vi "Parse and Attach Metadata to TDMS.vi"(8 "error in (no error)":errorcluster, 11 "experiment folder":path) -> (0 "error out":errorcluster, 2 "file path out":path)   [LabVIEW 2016]
uses:
  <userlib>/_OpenG.lib/file/file.llb/Build Path - Traditional__ogtk.vi
  <userlib>/LevyLab/LV to ITX/Data/Data.lvclass
panel:
  out "wiring":string[][][](array[string])
  out "itx notes parsed iterations":i32
  out "Array":string[](array[string])
  out "group/channel names":string[][](array[string])
  out "group names":string[](array[string])
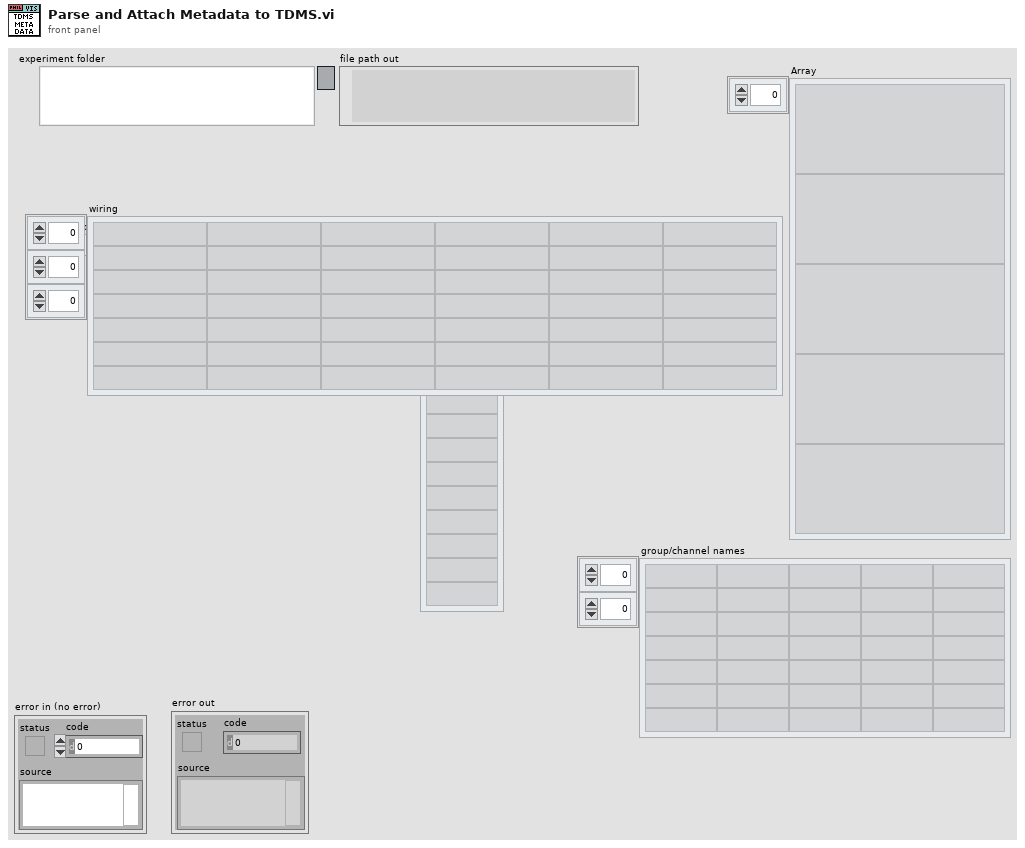
[diagram p1: front panel]
types:
  T1 = enum16{"open", "open or create", "create or replace", "create", "open (read-only)"}
  T2 = cluster{"Scan control":cluster{"Priority":enum16{"Priority 0", "Priority 1", "Priority 2", "Priority 3", "Priority 4", "Priority 5"}, "Scan name":enum16{"OFF", "DSA_Vsg2", "DSA_Vsg3", "DSA_Vbg", "DSA_Vsg1", "DSA_freq", "DSA_Vamp", "time", "Lockin Amplitude", "Lockin Frequency", "Lockin Bias", "Delay", "Strain", "DAQ Bias", "Magnet Field", "Temperature", "MW f1", "MW f2", "MW Amplitude1", "MW Amplitude2"}}[], "Scan parameters":cluster{"Start":dbl, "End":dbl, "Step":dbl, "Rate":dbl, "wait (ms)":u32, "Address":string, "channel":i32}[], "Experiment":enum16{"IV", "IV_Fast", "IV_Sweep", "THz_DelayLine", "Lockin_Vsg", "Lockin_Sweep", "Lockin_Time", "AI WFM time", "Lockin (experimental)"}}
  T3 = cluster{"AO Amp (V)":dbl[], "AO DC (V)":dbl[], "AO f (Hz)":dbl[], "AO Phase (°)":dbl[], "Function":enum16{"Sine", "Triangle", "Square", "Sawtooth"}[], "I+":bool[], "Sweeping":bool[]}
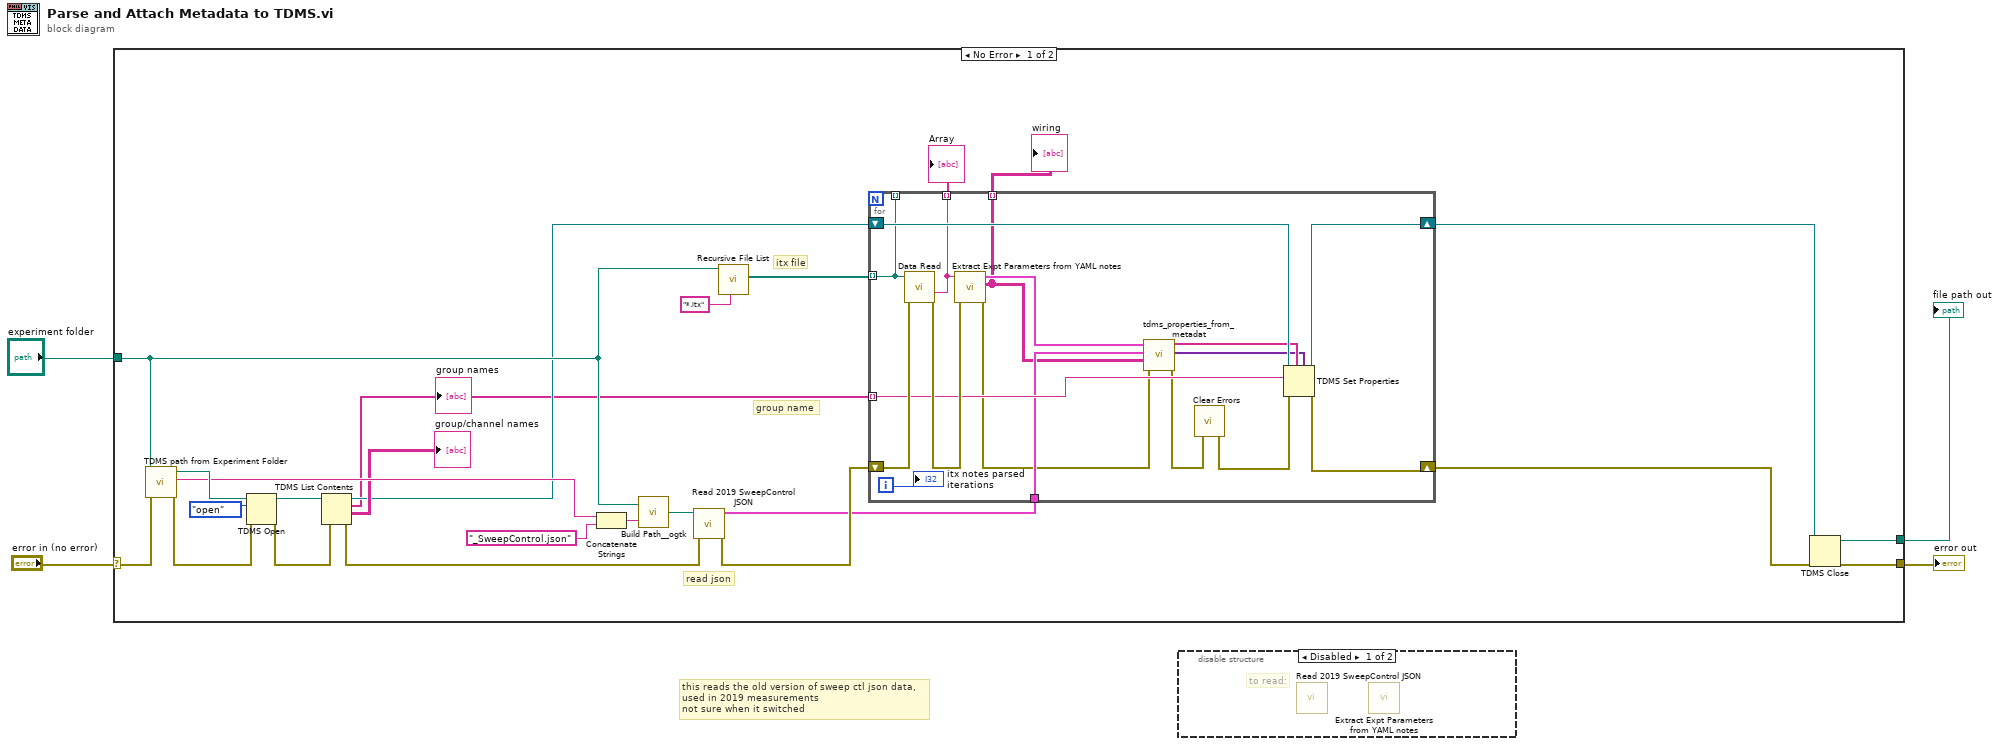
[diagram p0: block diagram]
diagram:
  # "this reads the old version of sweep ctl json data,\nused in 2019 measurements\nnot sure when it switched"
  n1 = case shown="No Error" "error in (no error)" {
    selector: "error in (no error)" -> [w25 w47]
    tunnel: [w12 w47] -> w3
    tunnel: "experiment folder" -> [w22 _]
    tunnel: [w11 _] -> w1
    frame No Error {
      # "itx file"
      # "group name"
      # "read json"
      n2 = call "TDMS path from Experiment Folder.vi"("error in (no error)"=w25, "experiment folder"=w22) -> ("error out"=w24:errorcluster, "name"=w21:string, "tdms file path"=w23:path)  [unwired: 7 in]
      n3 = TDMS Open(8:w24, 10:T1."open" ("operation (0:open)"), 11:w23) -> (0:w20:errorcluster, 3:w18:refnum<k34>)  [unwired: 4 in]
      n4 = TDMS List Contents(4:w20, 7:w18) -> (0:w13:errorcluster, 1:→"group/channel names":string[][], 2:w8:string[], 3:w14:refnum<k34>)  [unwired: 1 in]
      "group names" <- w8
      n5 = Concatenate Strings(w21, "_SweepControl.json" ("string")) -> (w28:string)
      n6 = call-poly <userlib>:"Build Path__ogtk.vi"("name or relative path"=w28, "base path"=w22) -> ("appended path"=w16:path)
      n7 = call "Read 2019 SweepControl JSON.vi"("error in (no error)"=w13, "json file"=w16) -> ("error out"=w15:errorcluster, "data"=w10:T2)  [unwired: 8 in]
      n8 = call <vilib>:"Recursive File List.vi"("pattern"="*.itx", "Folder Path"=w22) -> ("All Files in Dir"=w17:path[])  [unwired: 5 in, 4 out]
      n9 = for {
        tunnel: w17 -> [w35] mode=indexing
        shift-right: [w31] -> w6
        shift-left: w15 -> [w46]
        tunnel: w8 -> [w42] mode=indexing
        shift-right: [w43] -> w9
        shift-left: w14 -> [w44]
        tunnel: w10 -> [w41]
        tunnel: [w36] -> w7 mode=indexing
        tunnel: [w35] -> _ mode=indexing
        tunnel: [w30] -> w5 mode=indexing
        i -> [w34]
        n10 = call <userlib>:"Data Read.vi"("error in (no error)"=w46, "path"=w35) -> ("error out"=w45:errorcluster, "Notes"=w36:string)  [unwired: 6 in, 2 out]
        n11 = call "Extract Expt Parameters from YAML notes.vi"("error in (no error)"=w45, "YAML Comments IN"=w36) -> ("error out"=w37:errorcluster, "wiring"=w30:string[][], "Experiment Parameters From 1st ITX"=w40:T3)  [unwired: 6 in, 1 out]
        n12 = call "tdms_properties_from_metadat.vi"("error in (no error)"=w37, "wiring"=w30, "data"=w41, "Experiment Parameters From 1st ITX"=w40) -> ("error out"=w33:errorcluster, "property values"=w38:variant[], "property names"=w39:string[])  [unwired: 5 in]
        n13 = call <vilib>:"Clear Errors.vi"("error in (no error)"=w33) -> ("error out"=w32:errorcluster)  [unwired: 5 in, 1 out]
        n14 = TDMS Set Properties(5:w38, 7:w39, 8:w32, 10:w42, 11:w44) -> (0:w31:errorcluster, 3:w43:refnum<k34>)  [unwired: 1 in, 2 out]
        "itx notes parsed iterations" <- w34
      }
      "Array" <- w7
      "wiring" <- w5
      n15 = TDMS Close(8:w6, 11:w9) -> (0:w12:errorcluster, 3:w11:path)
    }
    frame Error {
    }
  }
  "error out" <- w3
  "file path out" <- w1
  n16 = disable-structure shown="Disabled" {
    frame Disabled {
      # "to read:"
      n17 = call "Read 2019 SweepControl JSON.vi"() -> ()  [unwired: 10 in, 2 out]
      n18 = call "Extract Expt Parameters from YAML notes.vi"() -> ()  [unwired: 8 in, 4 out]
    }
    frame Enabled {
    }
  }
